vi "To and From String Array.vi"() -> ()   [LabVIEW 2015, in "Update Tag Tests.lvlib"]
uses:
  Update Tag Tests.lvlib
  <vilib>/NI/Tag Bus/tag/Data Type.ctl
  Config/Update Tag Configuration/Update Tag Config.lvclass
  <vilib>/NI/Tag Bus Module Framework/channel/channel classification.ctl
  <vilib>/NI/Tag Bus/tag/tag descriptor.lvclass
  <vilib>/NI/Tag Bus Module Framework/channel/TBM channel.lvclass
panel:
  out "Second String Array":string[][](array[string])
  out "Origianl String Array":string[][](array[string])
  out "error out":errorcluster
  out "Pass":bool
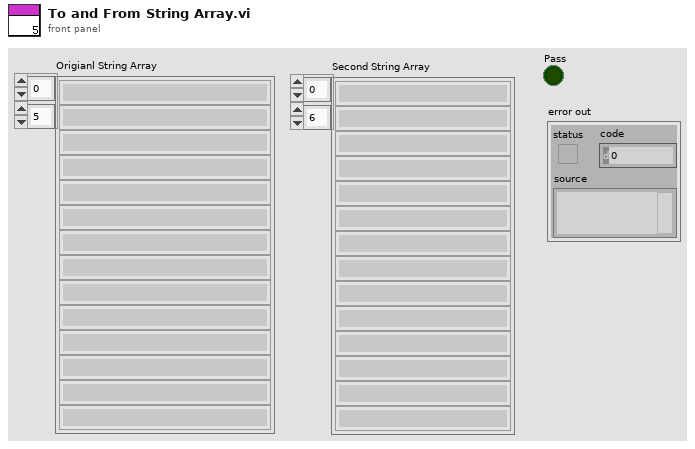
[diagram p1: front panel]
types:
  T1 = typedef "tag bus.lvlib/tag descriptor.lvclass/Data Type.ctl" = enum16{"Double", "Single", "I64", "I32", "I16", "I8", "U64", "U32", "U16", "U8", "Boolean", "String", "Array of Double", "Array of Single", "Array of I64", "Array of I32", "Array of I16", "Array of I8", "Array of U64", "Array of U32", "Array of U16", "Array of U8", "Array of Boolean", "Array of String"}
  T2 = typedef "TBM channel.lvclass/channel classification.ctl" = enum16{"input data", "output data", "processing parameter", "processing result"}
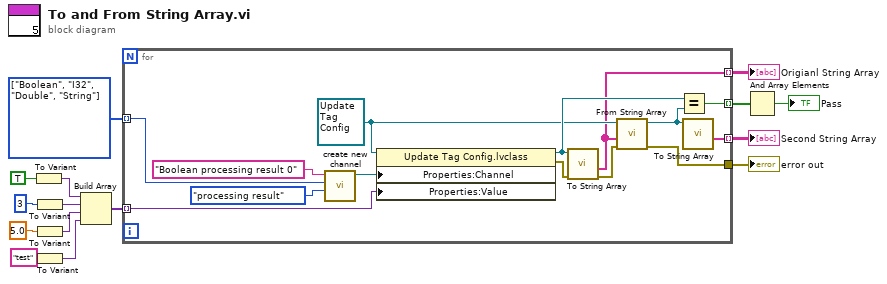
[diagram p0: block diagram]
diagram:
  w13 = T1[] [enum."Boolean", enum."I32", enum."Double", enum."String"] items=["Double", "Single", "I64", "I32", "I16", "I8", "U64", "U32", "U16", "U8", "Boolean", "String", "Array of Double", "Array of Single", "Array of I64", "Array of I32", "Array of I16", "Array of I8", "Array of U64", "Array of U32", "Array of U16", "Array of U8", "Array of Boolean", "Array of String"] ("Data Type")
  n1 = To Variant(anything=TRUE) -> (Variant=w12:variant)
  n2 = To Variant(anything=3) -> (Variant=w11:variant)
  n3 = To Variant(anything=5.0) -> (Variant=w10:variant)
  n4 = To Variant(anything="test") -> (Variant=w9:variant)
  n5 = Build Array(w12, w11, w10, w9) -> (w8:variant[])
  n6 = for {
    tunnel: [w23] -> w3 mode=indexing
    tunnel: [w22] -> w15
    tunnel: [w20] -> w14 mode=indexing
    tunnel: w13 -> [w19] mode=indexing
    tunnel: w8 -> [w18] mode=indexing
    tunnel: [w16] -> w1 mode=indexing
    w17 = refnum<class "Update Tag Config.lvclass"> refnum ("Update Tag Config.lvclass")
    n7 = call <vilib>:"create new channel.vi"("channel classification"=channel_classification."processing result", "data type"=w19, "channel name"="Boolean processing result 0" ("Tag Name 2")) -> ("channel"=w27:refnum<class "TBM channel.lvclass">)  [unwired: 8 in]
    n8 = property class="Update Tag Config.lvclass"(reference=w17, "Properties:Channel"=w27, "Properties:Value"=w18) -> (reference out=w24:refnum<class "Update Tag Config.lvclass">, error out=w26:errorcluster)  [unwired: 1 in]
    n9 = call-dynamic "To String Array.vi"("error in (no error)"=w26, "Update Tag Config in"=w24) -> ("error out"=w25:errorcluster, "Step String Array"=w16:string[])  [unwired: 7 in, 1 out]
    n10 = call-dynamic "From String Array.vi"("error in (no error)"=w25, "String Array"=w16, "Update Tag Config in"=w17) -> ("error out"=w22:errorcluster, "Update Tag Config out"=w21:refnum<class "Update Tag Config.lvclass">)  [unwired: 5 in, 2 out]
    n11 = Equal?(x=w24, y=w21) -> (x = y?=w23:bool)
    n12 = call-dynamic "To String Array.vi"("Update Tag Config in"=w21) -> ("Step String Array"=w20:string[])  [unwired: 8 in, 2 out]
  }
  "error out" <- w15
  "Second String Array" <- w14
  "Origianl String Array" <- w1
  n13 = And Array Elements(Boolean array=w3) -> (logical AND=→"Pass":bool)
